vi "Init.vi"(8 "error in (no error)":errorcluster, 11 "PsuVisaSim in":refnum<class "PsuVisaSim.lvclass">) -> (0 "error out":errorcluster, 3 "PsuVisaSim out":refnum<class "PsuVisaSim.lvclass">)   [LabVIEW 2020, in "LAF2024Q2.lvlib" / "PsuVisaSim.lvclass"]
uses:
  PsuVisaSim.lvclass
  C:/dev/lv 2020/laf-2024-q2/LAF2024Q2/PowerSupplyVisa/PowerSupplyVisa.lvclass
  C:/dev/lv 2020/laf-2024-q2/LAF2024Q2/PowerSupply/PowerSupply.lvclass
  PowerSupplyVisa/PowerSupplyVisa.lvclass
  PowerSupply/PowerSupply.lvclass
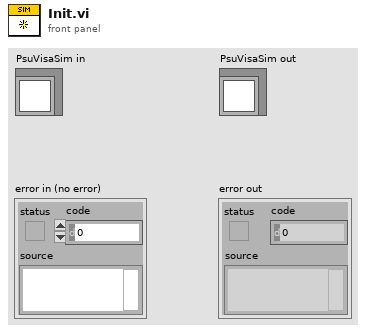
[diagram p1: front panel]
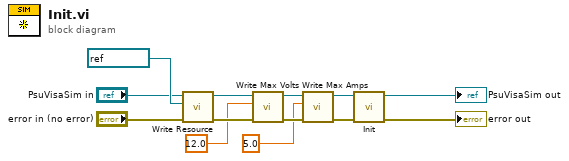
[diagram p0: block diagram]
diagram:
  n1 = call "Write Resource.vi"("error in (no error)"="error in (no error)", "Resource"=refnum<visa-resource-name> "COM2", "PowerSupplyVisa in"="PsuVisaSim in") -> ("error out"=w13:errorcluster, "PowerSupplyVisa out"=w11:refnum<class "PsuVisaSim.lvclass">)  [unwired: 7 in]
  n2 = call "Write Max Volts.vi"("error in (no error)"=w13, "Max Voltage"=12.0, "PowerSupply in"=w11) -> ("error out"=w7:errorcluster, "PowerSupply out"=w3:refnum<class "PsuVisaSim.lvclass">)  [unwired: 7 in]
  n3 = call "Write Max Amps.vi"("error in (no error)"=w7, "Max Current"=5.0 ("Max Voltage"), "PowerSupply in"=w3) -> ("error out"=w4:errorcluster, "PowerSupply out"=w2:refnum<class "PsuVisaSim.lvclass">)  [unwired: 7 in]
  n4 = call-parent "Init.vi"("error in (no error)"=w4, "PowerSupply in"=w2) -> ("error out"=→"error out":errorcluster, "PowerSupply out"=→"PsuVisaSim out":refnum<class "PsuVisaSim.lvclass">)  [unwired: 8 in]
